vi "Published Trace.vi"(8 "error in (no error)":errorcluster, 10 "Trace":refnum<class "Trace.lvclass">, 11 "Comp Trace Logger in":refnum<class "Comp Trace Logger.lvclass">) -> (0 "error out":errorcluster, 3 "Comp Trace Logger out":refnum<class "Comp Trace Logger.lvclass">)   [LabVIEW 2014, in "Comp Trace Logger.lvlib" / "Comp Trace Logger.lvclass"]
uses:
  Comp Trace Logger.lvclass
  Robot Actor Framework/Trace/Trace Class/Trace.lvclass
  Comp Trace Logger.lvclass/Comp Trace Logger.ctl
  Robot Actor Framework/Trace/Trace Listener Class/Trace Listener.lvclass
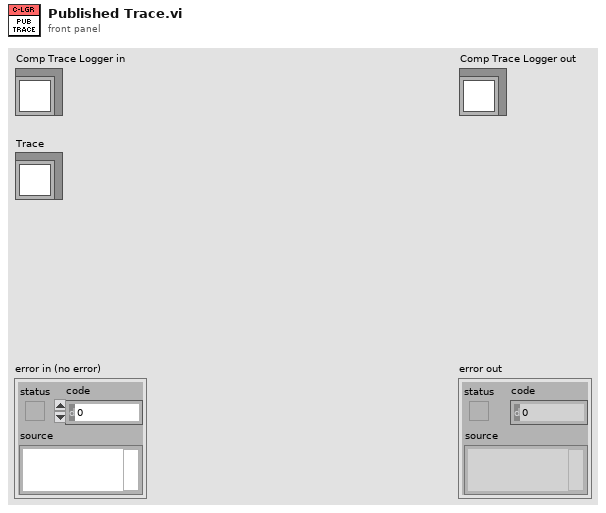
[diagram p1: front panel]
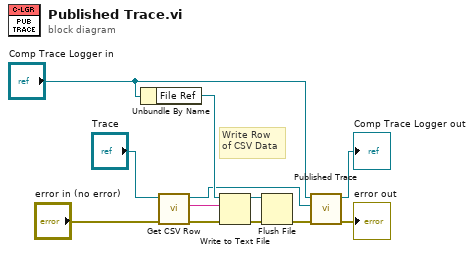
[diagram p0: block diagram]
diagram:
  # "Write Row\nof CSV Data"
  n1 = Unbundle By Name("Comp Trace Logger in") -> ("File Ref"=w9:refnum<file>)
  n2 = call-dynamic "Get CSV Row.vi"("error in (no error)"="error in (no error)", "Trace in"="Trace") -> ("error out"=w5:errorcluster, "CSV Row"=w7:string, "Trace out"=w4:refnum<class "Trace.lvclass">)  [unwired: 7 in]
  n3 = Write to Text File(file (use dialog)=w9, text=w7, error in=w5) -> (refnum out=w1:refnum<file>, error out=w3:errorcluster)  [unwired: 1 in, 1 out]
  n4 = Flush File(refnum=w1, error in=w3) -> (error out=w2:errorcluster)  [unwired: 1 out]
  n5 = call-parent "Published Trace.vi"("error in (no error)"=w2, "Trace"=w4, "Trace Listener in"="Comp Trace Logger in") -> ("error out"=→"error out":errorcluster, "Trace Listener out"=→"Comp Trace Logger out":refnum<class "Comp Trace Logger.lvclass">)  [unwired: 7 in]
